vi "plantillagraficassonidos.vi"() -> ()   [LabVIEW 2016]
panel:
  out "Gráficas juntas":waveform(dbl)[](graph)
  out "Gráfica del promedio":waveform(dbl)(graph)
  in  "Dirección inicial\n del archivo .wav":path
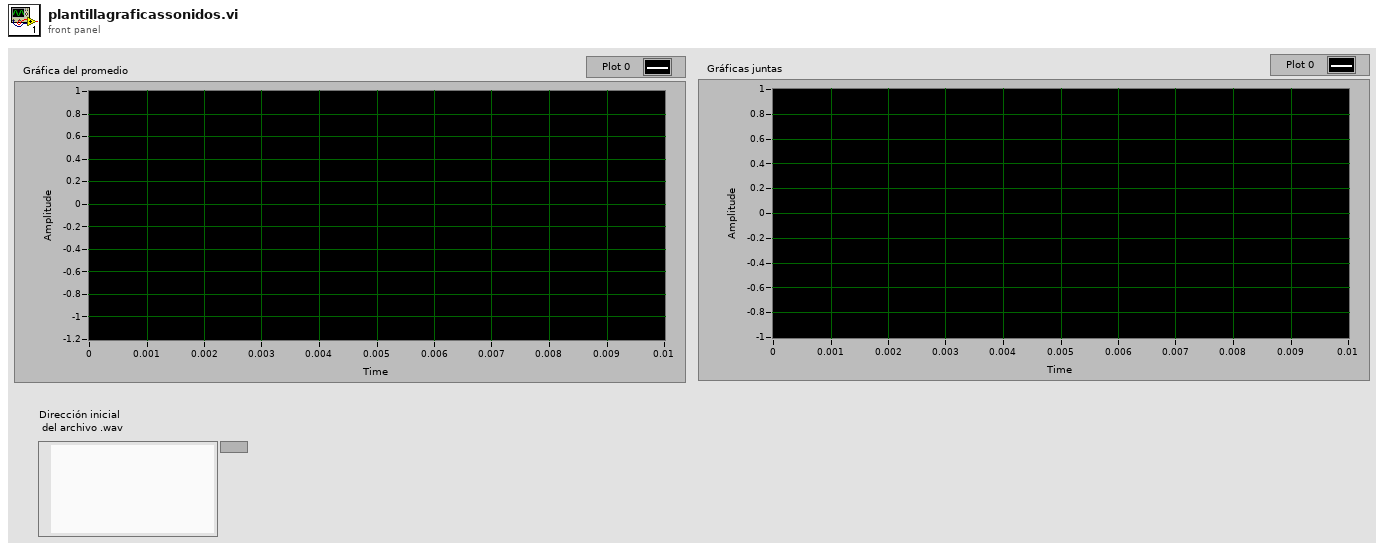
[diagram p1: front panel]
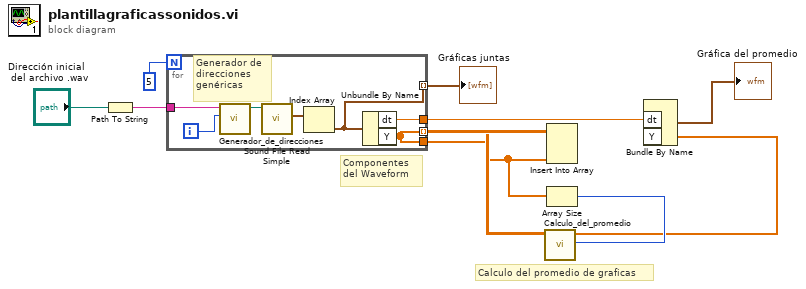
[diagram p0: block diagram]
diagram:
  # "Componentes \ndel Waveform"
  # "Calculo del promedio de graficas"
  n1 = Path To String(path="Dirección inicial\n del archivo .wav") -> (string=w9:string)
  n2 = for {
    N: 5 -> [_]
    tunnel: w9 -> [w16]
    tunnel: [w13] -> w7 mode=indexing
    tunnel: [w15] -> w8
    tunnel: [w13] -> w2
    tunnel: [w12] -> w1 mode=indexing
    i -> [w14]
    # "Generador de \ndirecciones \ngenéricas"
    n3 = call "Generador_de_direcciones.vi"("Numeric"=w14, "String"=w16) -> ("Path"=w17:path)  [unwired: 9 in]
    n4 = call <vilib>:"Sound File Read Simple.vi"("path"=w17) -> ("data"=w18:waveform(dbl)[])  [unwired: 7 in, 3 out]
    n5 = Index Array(array=w18) -> (element=w12:waveform(dbl))  [unwired: 1 in]
    n6 = Unbundle By Name(w12) -> ("dt"=w15:dbl, "Y"=w13:dbl[])
  }
  "Gráficas juntas" <- w1
  n7 = Insert Into Array(array=w7, new element=w2) -> (w5:dbl[][])  [unwired: 2 in]
  n8 = Array Size(array=w2) -> (size(s)=w6:i32)
  n9 = call "Calculo_del_promedio.vi"("Numeric"=w6, "Y"=w5) -> ("Array"=w4:dbl[])  [unwired: 9 in]
  n10 = Bundle By Name("dt"=w8, "Y"=w4) -> (→"Gráfica del promedio":waveform(dbl))  [unwired: 1 in]
